vi "3D Initialisation.vi"(11 "reference":refnum<vi>) -> (0 "Telescope":refnum<vi>, 1 "Gimbal":refnum<vi>, 2 "Base":refnum<vi>, 3 "Scene Object":refnum<vi>, 4 "error out":errorcluster)   [LabVIEW 2015]
uses:
  <vilib>/Utility/miscctls.llb/LV3DPointTypeDef.ctl
  <vilib>/picture/3D Picture Control/Object/Create Object (name).vi
  <vilib>/picture/3D Picture Control/Object/Add Object (no reference).vi
  <vilib>/picture/3D Picture Control/Object/Create Object (drawable).vi
  <vilib>/picture/3D Picture Control/Object/Add Object (reference).vi
  <vilib>/picture/3D Picture Control/NI_3D Picture Control.lvlib
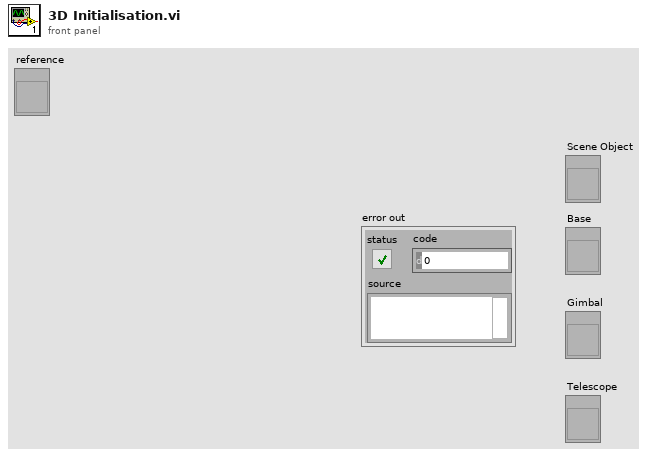
[diagram p1: front panel]
types:
  T1 = typedef "LV3DPointTypeDef.ctl" = cluster{"X":sgl, "Y":sgl, "Z":sgl}
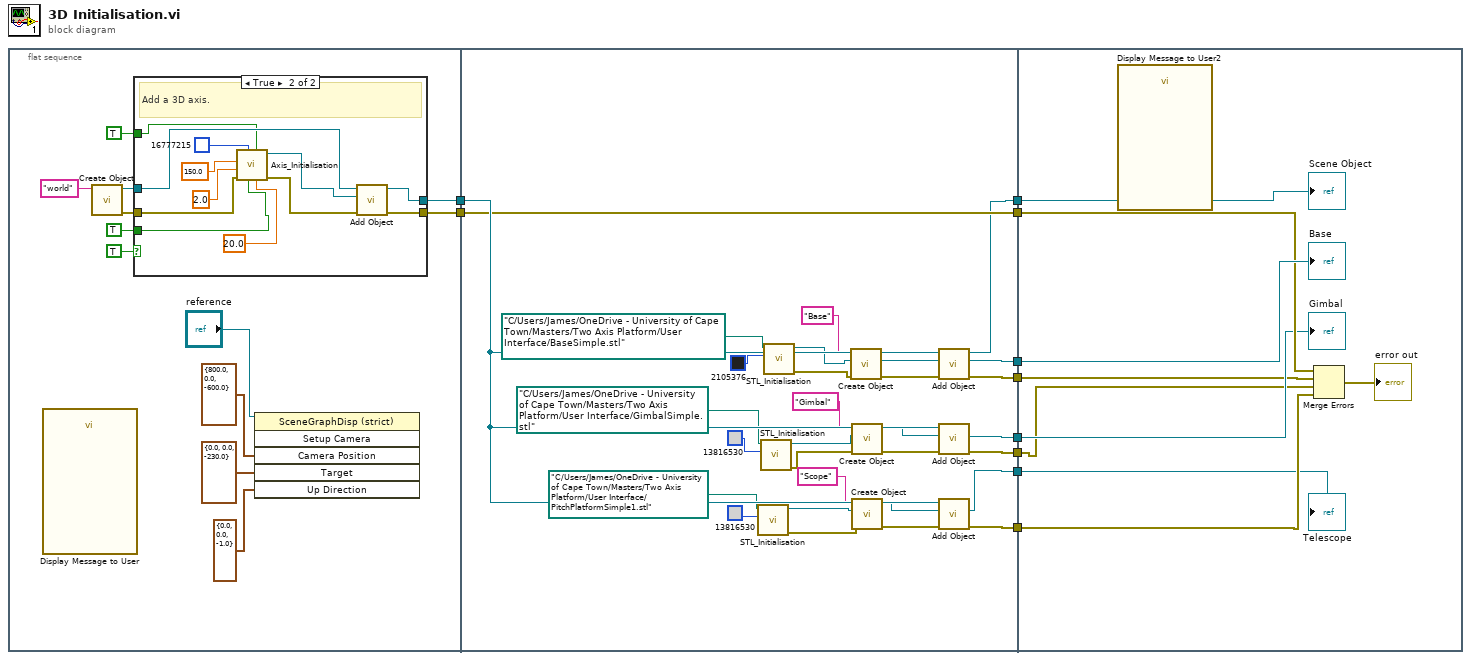
[diagram p0: block diagram]
diagram:
  n1 = flat-sequence {
    tunnel: [w17] -> w10
    tunnel: [w11] -> w9
    tunnel: w10 -> [w65]
    tunnel: w9 -> [w66]
    tunnel: [w65] -> w8
    tunnel: [w64] -> w7
    tunnel: [w63] -> w6
    tunnel: [w62] -> w5
    tunnel: [w61] -> w4
    tunnel: [w60] -> w3
    tunnel: [w59] -> w2
    tunnel: [w58] -> w1
    tunnel: w8 -> [w72]
    tunnel: w7 -> [w74]
    tunnel: w6 -> [w73]
    tunnel: w5 -> [w70]
    tunnel: w4 -> [w71]
    tunnel: w3 -> [w69]
    tunnel: w2 -> [w67]
    tunnel: w1 -> [w68]
    frame #0 {
      n2 = call "Display Message to User"() -> ()  [unwired: 10 in, 2 out]
      n3 = call-poly <vilib>:"Create Object.vi"("Name"="world") -> ("error out"=w22:errorcluster, "Scene:New Object"=w21:refnum<vi>)  [unwired: 9 in]
      n4 = case shown="True" TRUE ("show axis") {
        tunnel: [w24 w35] -> w11
        tunnel: TRUE ("Half plane?") -> [_ w32]
        tunnel: [w23 w34] -> w17
        tunnel: TRUE ("Axis label?") -> [_ w28]
        tunnel: w21 -> [w24 w36]
        tunnel: w22 -> [w23 w25]
        frame False {
          # "Pass an empty model when displaying no axis."
        }
        frame True {
          # "Add a 3D axis."
          n5 = call "Axis_Initialisation.vi"("Character Size"=sgl 20.0, "Half plane?"=w32, "Axis label?"=w28, "Color 2"=u32 16777215 ("Color"), "error in (no error)"=w25, "Radius"=sgl 2.0, "Length"=sgl 150.0 ("Height")) -> ("error out"=w30:errorcluster, "New Object Refnum"=w31:refnum<vi>)  [unwired: 3 in]
          n6 = call-poly <vilib>:"Add Object.vi"("error in (no error)"=w30, "New Object In"=w31, "Scene Object In"=w36) -> ("error out"=w34:errorcluster, "Scene Object Out"=w35:refnum<vi>)  [unwired: 7 in]
        }
      }
      n7 = invoke on="Invoke Node" class="SceneGraphDisp (strict)" method="Setup Camera"(reference="reference", "Camera Position"=T1 {"X"=800.0, "Y"=0.0, "Z"=-600.0}, "Target"=T1 {"X"=0.0, "Y"=0.0, "Z"=-230.0}, "Up Direction"=T1 {"X"=0.0, "Y"=0.0, "Z"=-1.0}) -> ()  [unwired: 2 in, 6 out]
    }
    frame #1 {
      n8 = call "STL_Initialisation.vi"("Color"=u32 13816530, "Model File"=path "C:/Users/James/OneDrive - University of Cape Town/Masters/Two Axis Platform/User Interface/PitchPlatformSimple1.stl" ("Telescope")) -> ("error out"=w39:errorcluster, "New Mesh Refnum"=w38:refnum<vi>)  [unwired: 8 in]
      n9 = call "STL_Initialisation.vi"("Color"=u32 13816530, "Model File"=path "C:/Users/James/OneDrive - University of Cape Town/Masters/Two Axis Platform/User Interface/GimbalSimple.stl" ("Gimbal")) -> ("error out"=w42:errorcluster, "New Mesh Refnum"=w43:refnum<vi>)  [unwired: 8 in]
      n10 = call "STL_Initialisation.vi"("Color"=u32 2105376, "Model File"=path "C:/Users/James/OneDrive - University of Cape Town/Masters/Two Axis Platform/User Interface/BaseSimple.stl" ("Base File")) -> ("error out"=w47:errorcluster, "New Mesh Refnum"=w46:refnum<vi>)  [unwired: 8 in]
      n11 = call-poly <vilib>:"Create Object.vi"("error in (no error)"=w47, "Geometry"=w46, "Name"="Base") -> ("error out"=w50:errorcluster, "Scene:New Object"=w53:refnum<vi>)  [unwired: 7 in]
      n12 = call-poly <vilib>:"Create Object.vi"("error in (no error)"=w42, "Geometry"=w43, "Name"="Gimbal") -> ("error out"=w51:errorcluster, "Scene:New Object"=w55:refnum<vi>)  [unwired: 7 in]
      n13 = call-poly <vilib>:"Create Object.vi"("error in (no error)"=w39, "Geometry"=w38, "Name"="Scope") -> ("error out"=w52:errorcluster, "Scene:New Object"=w54:refnum<vi>)  [unwired: 7 in]
      n14 = call-poly <vilib>:"Add Object.vi"("error in (no error)"=w50, "New Object In"=w53, "Scene Object In"=w66) -> ("error out"=w62:errorcluster, "New Object Out"=w63:refnum<vi>, "Scene Object Out"=w64:refnum<vi>)  [unwired: 6 in]
      n15 = call-poly <vilib>:"Add Object.vi"("error in (no error)"=w51, "New Object In"=w55, "Scene Object In"=w66) -> ("error out"=w60:errorcluster, "New Object Out"=w61:refnum<vi>)  [unwired: 6 in, 1 out]
      n16 = call-poly <vilib>:"Add Object.vi"("error in (no error)"=w52, "New Object In"=w54, "Scene Object In"=w66) -> ("error out"=w58:errorcluster, "New Object Out"=w59:refnum<vi>)  [unwired: 6 in, 1 out]
    }
    frame #2 {
      n17 = call "Display Message to User2"() -> ()  [unwired: 10 in, 2 out]
      n18 = Merge Errors(w72, w70, w69, w68) -> (→"error out":errorcluster)
      "Telescope" <- w67
      "Scene Object" <- w74
      "Base" <- w73
      "Gimbal" <- w71
    }
  }
